vi "CSM Module.vi"(7 "Name (\"\" to Use UUID)":string="CSM Tiny") -> ()   [LabVIEW 2017]
uses:
  src/user.lib/_NEVSTOP/Communicable State Machine(CSM)/AdvanceAPI/CSM - Revert Arguments-Safe String.vi
  src/user.lib/_NEVSTOP/Communicable State Machine(CSM)/AdvanceAPI/CSM - Make String Arguments Safe.vi
  src/user.lib/_NEVSTOP/Communicable State Machine(CSM)/AdvanceAPI/CSM - Break Down Multiple States String.vi
  src/user.lib/_NEVSTOP/Communicable State Machine(CSM)/AdvanceAPI/CSM - Compact Multiple States.vi
  src/user.lib/_NEVSTOP/Communicable State Machine(CSM)/AdvanceAPI/CSM - Keywords.vi
  src/user.lib/_NEVSTOP/Communicable State Machine(CSM)/_Shared/Trim Single-line Text.vi
  src/user.lib/_NEVSTOP/Communicable State Machine(CSM)/Communicable State Machine.lvlib
panel:
  out "State History":string
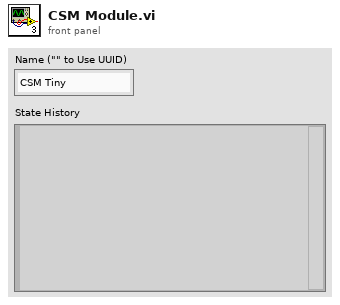
[diagram p1: front panel]
types:
  T1 = enum32{"Invalid", "Standard", "Closed", "Hidden", "Minimized", "Maximized"}
  T2 = enum32{"invalid app kind", "Development System", "Run Time System", "Student Edition", "Embedded LabVIEW", "Evaluation", "Custom"}
  T3 = typedef "Communicable State Machine.lvlib/_CSM_Response Source Message.ctl" = cluster{"‘State":string, "’Arguments":string, "’Error":errorcluster}
  T4 = cluster{"Current VI Reference":refnum<vi>, "Close Panel on Exit?":bool}
  T5 = cluster{"Core":cluster{"Current VI Reference":refnum<vi>, "Close Panel on Exit?":bool}, "Your Boolean data":bool, "Your string data":string}
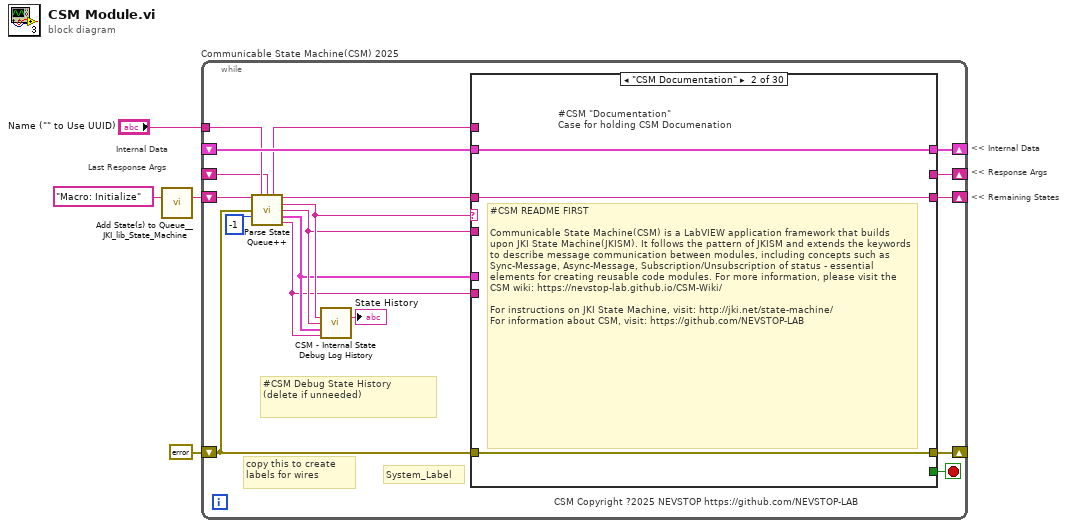
[diagram p0: block diagram]
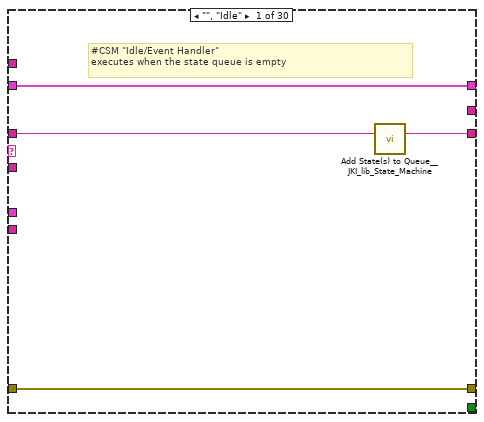
[diagram p2: hidden frame]
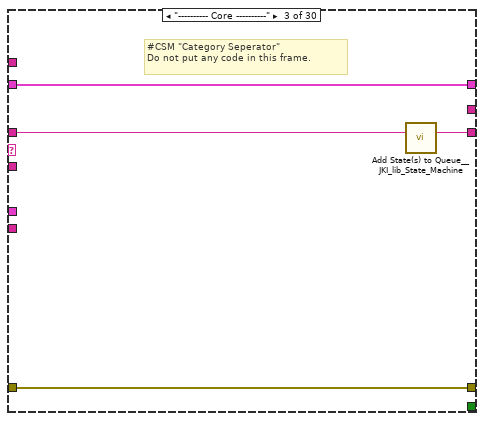
[diagram p3: hidden frame]
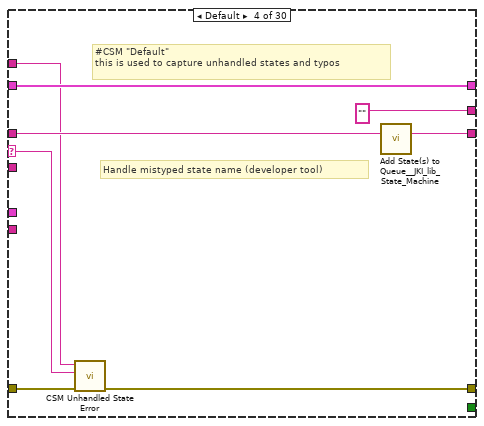
[diagram p4: hidden frame]
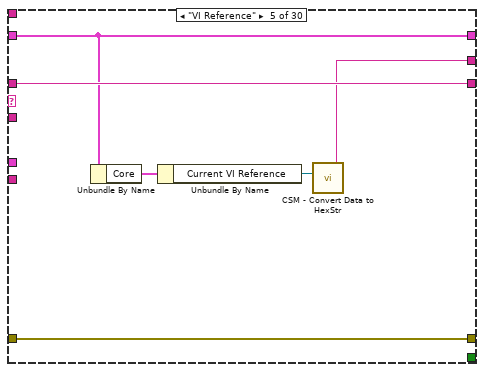
[diagram p5: hidden frame]
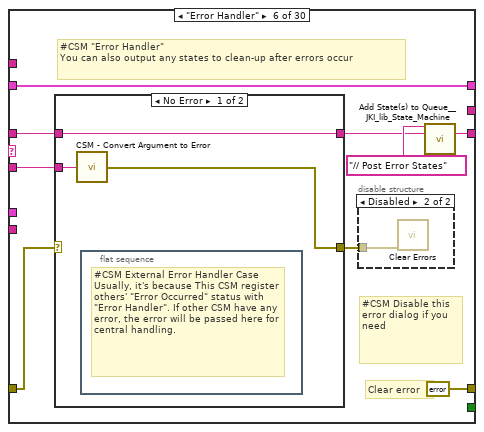
[diagram p6: hidden frame]
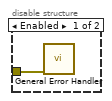
[diagram p7: hidden frame]
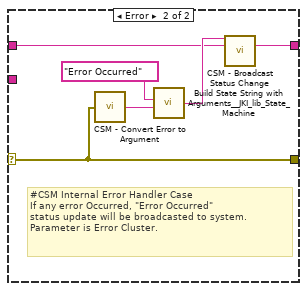
[diagram p8: hidden frame]
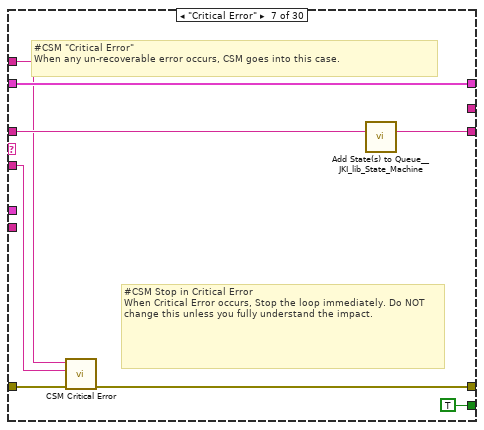
[diagram p9: hidden frame]
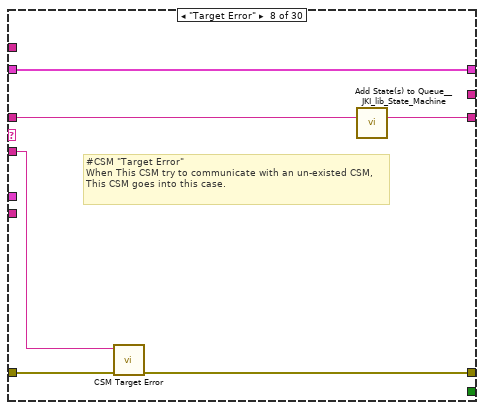
[diagram p10: hidden frame]
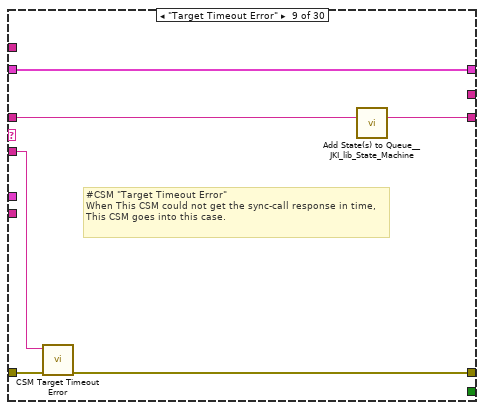
[diagram p11: hidden frame]
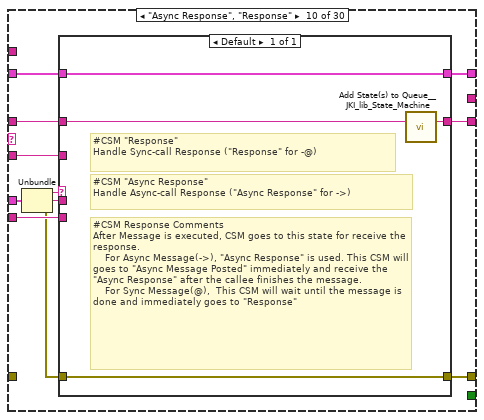
[diagram p12: hidden frame]
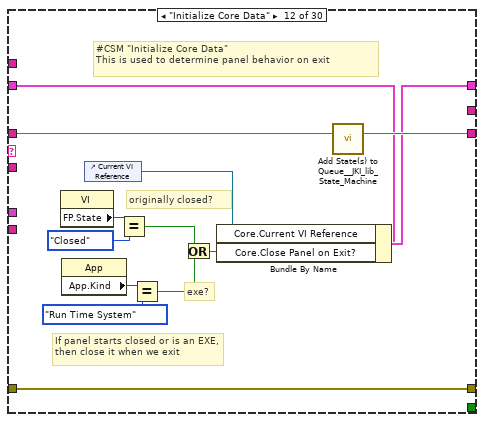
[diagram p14: hidden frame]
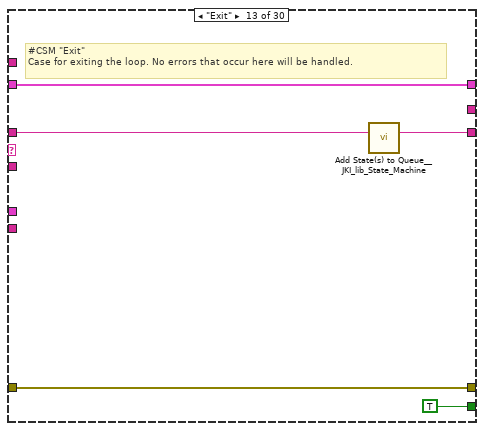
[diagram p15: hidden frame]
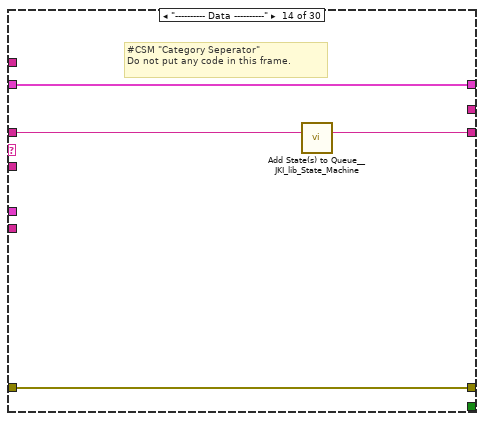
[diagram p16: hidden frame]
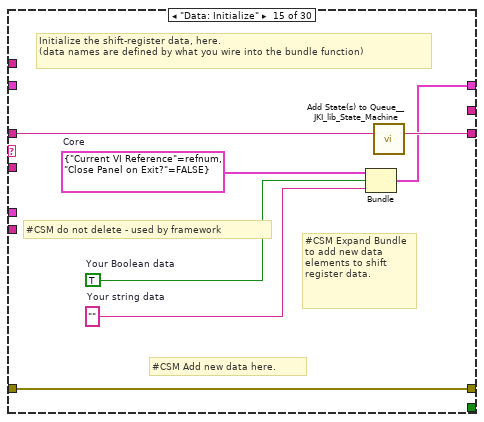
[diagram p17: hidden frame]
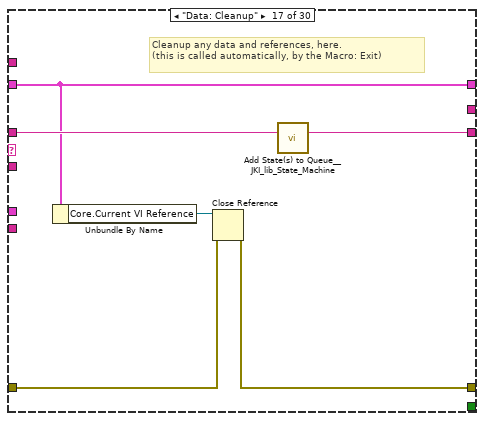
[diagram p19: hidden frame]
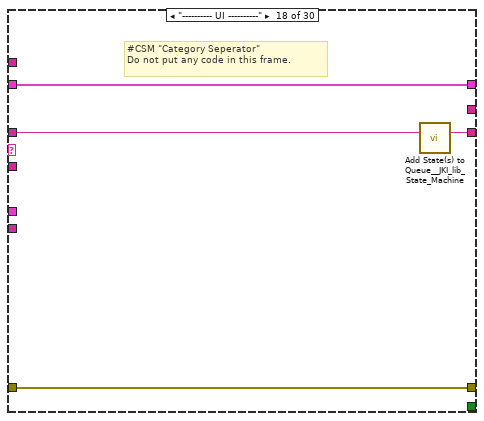
[diagram p20: hidden frame]
diagram:
  # "Last Response Args"
  # "Internal Data"
  # "<< Internal Data"
  # "<< Response Args"
  # "<< Remaining States"
  n1 = call <vilib>:"Add State(s) to Queue__JKI_lib_State_Machine.vi"("State(s) in (\"\")"="Macro: Initialize" ("Init State(\"Macro: Initialize\")")) -> ("States Out"=w4:string)  [unwired: 14 in]
  n2 = while "Communicable State Machine(CSM) 2025" {
    shift-right: [w17] -> _
    shift-left: _ -> [w16]
    shift-right: [w20] -> _
    shift-left: errorcluster {"status"=FALSE, "code"=0, "source"=""} ("error out") -> [w15]
    shift-right: [w19] -> _
    shift-left: w4 -> [w21]
    tunnel: "Name (\"\" to Use UUID)" -> [w13]
    shift-right: [w14] -> _
    shift-left: _ -> [w7]
    stop <- w18 stop-if-true
    # "#CSM Debug State History\n(delete if unneeded)"
    # "copy this to create labels for wires"
    # "System_Label"
    # "CSM Copyright ?2025 NEVSTOP https://github.com/NEVSTOP-LAB"
    n3 = call "Parse State Queue++.vi"("State Queue"=w21, "Name (\"\" to Use UUID)"=w13, "Response Arguments"=w7, "Previous Error"=w15, "Dequeue (1 ms)"=-1 ("Timeout")) -> ("Name Used"=w8:string, "Remaining States"=w22:string, "Current State"=w12:string, "Arguments"=w11:string, "Additional Information"=w10:T3, "Source CSM"=w9:string)  [unwired: 5 in]
    n4 = call "CSM - Internal State Debug Log History.vi"("State"=w12, "Arguments (\"\")"=w11, ">> Response Source Message >>"=w10, "Source (\"\")"=w9) -> ("Debug Log"=→"State History":string)  [unwired: 11 in]
    n5 = case shown="\"CSM Documentation\"" w12 {
      selector: w12 -> [_ _ _ w36 _ _ _ _ _ _ _ _ _ _ _ _ _ _ _ _ _ _ _ _ _ _ _ _ _ _]
      tunnel: w22 -> [w23 w28 w33 w40 w46 w52 w73 w79 w85 w93 w104 w118 w123 w127 w134 w136 w143 w147 w151 w157 w172 w241 w246 w253 w255 w259 w264 w271 w275 w279]
      tunnel: w11 -> [_ _ _ _ _ w51 w69 w78 w83 w92 _ _ _ _ _ _ _ _ _ w152 w166 _ _ _ _ _ w262 _ _ _]
      tunnel: w16 -> [w24 w27 w30 w38 w45 w55 w74 w80 w86 w95 w103 w111 w121 w124 _ w135 w138 w144 w149 w155 w168 w238 w243 w250 w254 w258 w263 w268 w272 w276]
      tunnel: [w25 w29 w31 w34 w47 errorcluster {"status"=FALSE, "code"=0, "source"=""} ("error out") w70 w76 w82 w98 w105 w115 w120 w125 w131 w137 w139 w145 w148 w153 w169 w239 w244 w251 w256 w260 w265 w269 w273 w277] -> w20
      tunnel: w15 -> [w25 w29 w31 w41 w47 w53 w75 w77 w84 _ w105 w115 w120 w125 w131 w137 w140 w145 w148 w154 w170 w239 w244 w251 w256 w260 w265 w269 w273 w277]
      tunnel: [w26 w28 w32 w39 w46 w48 w72 w81 w87 w94 w104 w117 w122 w126 w133 w136 w142 w146 w150 w156 w171 w240 w245 w252 w255 w259 w264 w270 w274 w278] -> w19
      tunnel: [_ _ _ _ _ _ TRUE _ _ _ _ _ TRUE _ _ _ _ _ _ _ _ _ _ _ _ _ _ _ _ _] -> w18
      tunnel: [w24 w27 w30 w38 w45 w55 w74 w80 w86 w96 w103 w116 w121 w124 w132 w135 w138 w144 w149 w155 w168 w238 w243 w250 w254 w258 w263 w268 w272 w276] -> w17
      tunnel: w9 -> [_ _ _ _ _ _ _ _ _ w90 _ _ _ _ _ _ _ _ _ _ _ _ _ _ _ _ _ _ _ _]
      tunnel: w10 -> [_ _ _ _ _ _ _ _ _ w97 _ _ _ _ _ _ _ _ _ _ _ _ _ _ _ _ _ _ _ _]
      tunnel: [_ _ _ "" w42 _ _ _ _ _ _ _ _ _ _ _ _ _ _ _ _ _ _ _ _ "API1 Response" w261 _ _ _] -> w14
      tunnel: w8 -> [_ _ _ w35 _ _ w68 _ _ _ _ _ _ _ _ _ _ _ _ _ _ _ _ _ _ _ _ _ _ _]
      frame "", "Idle" {
        # "#CSM \"Idle/Event Handler\"\nexecutes when the state queue is empty"
        n6 = call <vilib>:"Add State(s) to Queue__JKI_lib_State_Machine.vi"("State(s) in (\"\")"=w23) -> ("States Out"=w26:string)  [unwired: 14 in]
      }
      frame "CSM Documentation" {
        # "#CSM README FIRST\n\nCommunicable State Machine(CSM) is a LabVIEW application framework that builds upon JKI State Machine(JKISM). It follows the pattern of JKISM and extends the keywords to describe message communication between modules, including concepts such as Sync-Message, Async-Message, Subscription/Unsubscription of status - essential elements for creating reusable code modules. For more information, please visit the CSM wiki: https://nevstop-lab.github.io/CSM-Wiki/\n\nFor instructions on JKI State Machine, visit: http://jki.net/state-machine/\nFor information about CSM, visit: https://github.com/NEVSTOP-LAB"
        # "#CSM \"Documentation\"\nCase for holding CSM Documenation"
      }
      frame "---------- Core ----------" {
        # "#CSM \"Category Seperator\"\nDo not put any code in this frame."
        n7 = call <vilib>:"Add State(s) to Queue__JKI_lib_State_Machine.vi"("State(s) in (\"\")"=w33) -> ("States Out"=w32:string)  [unwired: 14 in]
      }
      frame Default {
        # "#CSM \"Default\"\nthis is used to capture unhandled states and typos"
        # "Handle mistyped state name (developer tool)"
        n8 = call "CSM Unhandled State Error.vi"("error in (no error)"=w41, "Undefined State"=w36, "CSM Name"=w35) -> ("error out"=w34:errorcluster)  [unwired: 8 in]
        n9 = call <vilib>:"Add State(s) to Queue__JKI_lib_State_Machine.vi"("State(s) in (\"\")"=w40) -> ("States Out"=w39:string)  [unwired: 14 in]
      }
      frame "VI Reference" {
        n10 = Unbundle By Name(w45) -> ("Core"=w44:T4)
        n11 = Unbundle By Name(w44) -> ("Current VI Reference"=w43:refnum<vi>)
        n12 = call "CSM - Convert Data to HexStr.vi"("Variant"=w43) -> ("HEX String (0-9,A-F)"=w42:string)  [unwired: 8 in]
      }
      frame "Error Handler" {
        # "#CSM Disable this error dialog if you need"
        # "#CSM \"Error Handler\"\nYou can also output any states to clean-up after errors occur"
        # "Clear error"
        n13 = case shown="No Error" w53 {
          selector: w53 -> [_ w62]
          tunnel: [w61 w64] -> w49
          tunnel: w52 -> [w61 w63]
          tunnel: w51 -> [w60 _]
          tunnel: [w59 w62] -> w54
          frame No Error {
            n14 = call "CSM - Convert Argument to Error.vi"("Argument"=w60) -> ("Error"=w59:errorcluster)  [unwired: 4 in]
            n15 = flat-sequence {
              frame #0 {
                # "#CSM External Error Handler Case\nUsually, it's because This CSM register others' \"Error Occurred\" status with \"Error Handler\". If other CSM have any error, the error will be passed here for central handling."
              }
            }
          }
          frame Error {
            # "#CSM Internal Error Handler Case \nIf any error Occurred, \"Error Occurred\" \nstatus update will be broadcasted to system.\nParameter is Error Cluster."
            n16 = call "CSM - Convert Error to Argument.vi"("Error"=w62) -> ("Argument"=w66:string)  [unwired: 4 in]
            n17 = call <vilib>:"Build State String with Arguments__JKI_lib_State_Machine.vi"("Arguments (\"\")"=w66, "State"="Error Occurred" ("Status with Arguments")) -> ("State with Arguments"=w65:string)  [unwired: 4 in]
            n18 = call "CSM - Broadcast Status Change.vi"("Status With Arguments"=w65, "State Queue"=w63) -> ("Remaining States"=w64:string)  [unwired: 13 in]
          }
        }
        n19 = disable-structure shown="Disabled" {
          disable-tunnel: w54 -> [w57 w58]
          frame Enabled {
            n20 = call <vilib>:"General Error Handler.vi"("error in (no error)"=w57) -> ()  [unwired: 10 in, 5 out]
          }
          frame Disabled {
            n21 = call <vilib>:"Clear Errors.vi"("error in (no error)"=w58) -> ()  [unwired: 5 in, 2 out]
          }
        }
        n22 = call <vilib>:"Add State(s) to Queue__JKI_lib_State_Machine.vi"("State(s) in Front (\"\")"="// Post Error States", "State(s) in (\"\")"=w49) -> ("States Out"=w48:string)  [unwired: 13 in]
      }
      frame "Critical Error" {
        # "#CSM Stop in Critical Error\nWhen Critical Error occurs, Stop the loop immediately. Do NOT change this unless you fully understand the impact."
        # "#CSM \"Critical Error\"\nWhen any un-recoverable error occurs, CSM goes into this case."
        n23 = call "CSM Critical Error.vi"("error in (no error)"=w75, "Arugments (As Reason)"=w69, "CSM Name"=w68) -> ("error out"=w70:errorcluster)  [unwired: 8 in]
        n24 = call <vilib>:"Add State(s) to Queue__JKI_lib_State_Machine.vi"("State(s) in (\"\")"=w73) -> ("States Out"=w72:string)  [unwired: 14 in]
      }
      frame "Target Error" {
        # "#CSM \"Target Error\"\nWhen This CSM try to communicate with an un-existed CSM, This CSM goes into this case."
        n25 = call "CSM Target Error.vi"("error in (no error)"=w77, "Arguments (As CSM Name)"=w78) -> ("error out"=w76:errorcluster)  [unwired: 9 in]
        n26 = call <vilib>:"Add State(s) to Queue__JKI_lib_State_Machine.vi"("State(s) in (\"\")"=w79) -> ("States Out"=w81:string)  [unwired: 14 in]
      }
      frame "Target Timeout Error" {
        # "#CSM \"Target Timeout Error\"\nWhen This CSM could not get the sync-call response in time, This CSM goes into this case."
        n27 = call "CSM Target Timeout Error.vi"("error in (no error)"=w84, "Arguments (As CSM Name)"=w83) -> ("error out"=w82:errorcluster)  [unwired: 9 in]
        n28 = call <vilib>:"Add State(s) to Queue__JKI_lib_State_Machine.vi"("State(s) in (\"\")"=w85) -> ("States Out"=w87:string)  [unwired: 14 in]
      }
      frame "Async Response", "Response" {
        n29 = Unbundle(w97) -> ("‘State"=w91:string, "’Arguments"=w89:string, "’Error"=w88:errorcluster)
        n30 = case shown="Default" w91 {
          tunnel: [w102] -> w98
          tunnel: w88 -> [w102]
          tunnel: [w101] -> w96
          tunnel: w95 -> [w101]
          tunnel: [w99] -> w94
          tunnel: w93 -> [w100]
          tunnel: w92 -> [_]
          tunnel: w90 -> [_]
          tunnel: w89 -> [_]
          frame Default {
            # "#CSM Response Comments\nAfter Message is executed, CSM goes to this state for receive the response.\n    For Async Message(->), \"Async Response\" is used. This CSM will goes to \"Async Message Posted\" immediately and receive the \"Async Response\" after the callee finishes the message.\n    For Sync Message(@),  This CSM will wait until the message is done and immediately goes to \"Response\""
            # "#CSM \"Async Response\"\nHandle Async-call Response (\"Async Response\" for ->)"
            # "#CSM \"Response\"\nHandle Sync-call Response (\"Response\" for -@)"
            n31 = call <vilib>:"Add State(s) to Queue__JKI_lib_State_Machine.vi"("State(s) in (\"\")"=w100) -> ("States Out"=w99:string)  [unwired: 14 in]
          }
        }
      }
      frame "Async Message Posted" {
        # "#CSM \"Async Message Posted\"\nAfter Async Message is posted (-> or ->| ), CSM goes to this state for post-action.\nYou can use Argument - State to tell which Async Message is called."
      }
      frame "Initialize Core Data" {
        # "#CSM \"Initialize Core Data\"\nThis is used to determine panel behavior on exit"
        # "originally closed?"
        # "exe?"
        # "If panel starts closed or is an EXE, then close it when we exit"
        n32 = property class="VI"() -> ("FP.State"=w108:T1)  [unwired: 2 in, 2 out]
        n33 = property class="App"() -> ("App.Kind"=w114:T2)  [unwired: 2 in, 2 out]
        n34 = control-ref of="Current VI Reference"() -> (w109:refnum<vi>)
        n35 = Equal?(x=w108, y=T1."Closed" ("Front Panel Window:State")) -> (x = y?=w106:bool)
        n36 = Equal?(x=w114, y=T2."Run Time System" ("Application:Kind")) -> (x = y?=w112:bool)
        n37 = Or(x=w106, y=w112) -> (x .or. y?=w110:bool)
        n38 = Bundle By Name(cluster=w111, "Core.Current VI Reference"=w109, "Core.Close Panel on Exit?"=w110) -> (w116:T5)
        n39 = call <vilib>:"Add State(s) to Queue__JKI_lib_State_Machine.vi"("State(s) in (\"\")"=w118) -> ("States Out"=w117:string)  [unwired: 14 in]
      }
      frame "Exit" {
        # "#CSM \"Exit\"\nCase for exiting the loop. No errors that occur here will be handled."
        n40 = call <vilib>:"Add State(s) to Queue__JKI_lib_State_Machine.vi"("State(s) in (\"\")"=w123) -> ("States Out"=w122:string)  [unwired: 14 in]
      }
      frame "---------- Data ----------" {
        # "#CSM \"Category Seperator\"\nDo not put any code in this frame."
        n41 = call <vilib>:"Add State(s) to Queue__JKI_lib_State_Machine.vi"("State(s) in (\"\")"=w127) -> ("States Out"=w126:string)  [unwired: 14 in]
      }
      frame "Data: Initialize" {
        w128 = T4 {"Current VI Reference"=refnum, "Close Panel on Exit?"=FALSE}  # Core
        w130 = TRUE  # Your Boolean data
        w129 = ""  # Your string data
        # "#CSM do not delete - used by framework"
        # "#CSM Expand Bundle to add new data elements to shift register data."
        # "#CSM Add new data here."
        # "Initialize the shift-register data, here.\n(data names are defined by what you wire into the bundle function)"
        n42 = Bundle("Core"=w128, "Your Boolean data"=w130, "Your string data"=w129) -> (w132:T5)  [unwired: 1 in]
        n43 = call <vilib>:"Add State(s) to Queue__JKI_lib_State_Machine.vi"("State(s) in (\"\")"=w134) -> ("States Out"=w133:string)  [unwired: 14 in]
      }
      frame "Data: Update Indicators" {
      }
      frame "Data: Cleanup" {
        # "Cleanup any data and references, here.\n(this is called automatically, by the Macro: Exit)"
        n44 = Unbundle By Name(w138) -> ("Core.Current VI Reference"=w141:refnum<vi>)
        n45 = Close Reference(reference=w141, error in (no error)=w140) -> (error out=w139:errorcluster)
        n46 = call <vilib>:"Add State(s) to Queue__JKI_lib_State_Machine.vi"("State(s) in (\"\")"=w143) -> ("States Out"=w142:string)  [unwired: 14 in]
      }
      frame "---------- UI ----------" {
        # "#CSM \"Category Seperator\"\nDo not put any code in this frame."
        n47 = call <vilib>:"Add State(s) to Queue__JKI_lib_State_Machine.vi"("State(s) in (\"\")"=w147) -> ("States Out"=w146:string)  [unwired: 14 in]
      }
      frame "UI: Initialize" {
        # "#CSM \"UI: Initialize\"\nInitialize the User Interface, here.\n(this is called automatically, by the Macro: Init)"
        n48 = call <vilib>:"Add State(s) to Queue__JKI_lib_State_Machine.vi"("State(s) in (\"\")"=w151) -> ("States Out"=w150:string)  [unwired: 14 in]
      }
      frame "UI: Cursor Set" {
        # "#CSM \"UI: Cursor Set\"\nSet and Unset Cursor Busy.\n(Usage: \"UI: Cursor Set >> Busy|Idle\")"
        # "Argument"
        n49 = disable-structure shown="TARGET_TYPE!=Windows" {
          disable-tunnel: w154 -> [w160 w165]
          disable-tunnel: [w159 w165] -> w153
          disable-tunnel: w152 -> [w158 _]
          frame condition #0 (active) {
            n50 = case shown="\"Idle\", Default" w158 {
              tunnel: w160 -> [w162 w164]
              tunnel: [w161 w163] -> w159
              frame "Idle", Default {
                n51 = call <vilib>:"Unset Busy.vi"("error in (no error)"=w162) -> ("error out"=w161:errorcluster)  [unwired: 10 in]
              }
              frame "Busy" {
                n52 = call <vilib>:"Set Busy.vi"("error in (no error)"=w164) -> ("error out"=w163:errorcluster)  [unwired: 9 in, 1 out]
              }
            }
          }
          frame condition #1 {
          }
        }
        n53 = call <vilib>:"Add State(s) to Queue__JKI_lib_State_Machine.vi"("State(s) in (\"\")"=w157) -> ("States Out"=w156:string)  [unwired: 14 in]
      }
      frame "UI: Front Panel State" {
        # "#CSM \"UI: Front Panel State\"\nSet Front Panel Open or Closed\n(Usage: \"UI: Front Panel State >> Open|Close\")"
        # "Argument"
        n54 = Unbundle By Name(w168) -> ("Core.Current VI Reference"=w167:refnum<vi>)
        n55 = call <vilib>:"Add State(s) to Queue__JKI_lib_State_Machine.vi"("State(s) in (\"\")"=w172) -> ("States Out"=w171:string)  [unwired: 14 in]
        n56 = case shown="\"Close\", \"Closed\"" w166 {
          tunnel: w170 -> [w178 w193 w204 w217 w230]
          tunnel: [w180 w194 w206 w219 w232] -> w169
          tunnel: w167 -> [w179 w191 w205 w218 w231]
          frame "Open", "Standard", Default {
            w173 = T1."Standard" ("State")
            n57 = property class="VI"(reference=w179, error in=w178) -> (reference out=w176:refnum<vi>, error out=w177:errorcluster, "FP.State"=w175:T1)
            n58 = Not Equal?(x=w175, y=w173) -> (x != y?=w174:bool)
            n59 = case shown="True" w174 {
              tunnel: [w184 w186] -> w180
              tunnel: w177 -> [w183 w186]
              tunnel: w176 -> [w182 _]
              tunnel: w173 -> [w181 _]
              frame True {
                n60 = invoke class="VI" method="FP.Open"(reference=w182, error in=w183, "Activate"=TRUE, "State"=w181) -> (error out=w184:errorcluster)  [unwired: 1 in, 4 out]
              }
              frame False {
              }
            }
          }
          frame "Close", "Closed" {
            n61 = property class="VI"(reference=w191, error in=w193) -> (reference out=w190:refnum<vi>, error out=w192:errorcluster, "FP.State"=w188:T1)
            n62 = Not Equal?(x=w188, y=T1."Closed" ("Front Panel Window:State")) -> (x != y?=w187:bool)
            n63 = case shown="False" w187 {
              tunnel: [w195 w198] -> w194
              tunnel: w192 -> [w195 w197]
              tunnel: w190 -> [_ w196]
              frame False {
              }
              frame True {
                n64 = invoke class="VI" method="FP.Close"(reference=w196, error in=w197) -> (error out=w198:errorcluster)  [unwired: 1 in, 2 out]
              }
            }
          }
          frame "Hidden", "Hide" {
            w199 = T1."Hidden" ("State")
            n65 = property class="VI"(reference=w205, error in=w204) -> (reference out=w202:refnum<vi>, error out=w203:errorcluster, "FP.State"=w201:T1)
            n66 = Not Equal?(x=w201, y=w199) -> (x != y?=w200:bool)
            n67 = case shown="True" w200 {
              tunnel: [w210 w211] -> w206
              tunnel: w203 -> [w209 w211]
              tunnel: w202 -> [w208 _]
              tunnel: w199 -> [w207 _]
              frame True {
                n68 = invoke class="VI" method="FP.Open"(reference=w208, error in=w209, "State"=w207) -> (error out=w210:errorcluster)  [unwired: 2 in, 4 out]
              }
              frame False {
              }
            }
          }
          frame "Minimize", "Minimized" {
            w212 = T1."Minimized" ("State")
            n69 = property class="VI"(reference=w218, error in=w217) -> (reference out=w215:refnum<vi>, error out=w216:errorcluster, "FP.State"=w214:T1)
            n70 = Not Equal?(x=w214, y=w212) -> (x != y?=w213:bool)
            n71 = case shown="True" w213 {
              tunnel: [w223 w224] -> w219
              tunnel: w216 -> [w222 w224]
              tunnel: w215 -> [w221 _]
              tunnel: w212 -> [w220 _]
              frame True {
                n72 = invoke class="VI" method="FP.Open"(reference=w221, error in=w222, "State"=w220) -> (error out=w223:errorcluster)  [unwired: 2 in, 4 out]
              }
              frame False {
              }
            }
          }
          frame "Maximize", "Maximized" {
            w225 = T1."Maximized" ("State")
            n73 = property class="VI"(reference=w231, error in=w230) -> (reference out=w228:refnum<vi>, error out=w229:errorcluster, "FP.State"=w227:T1)
            n74 = Not Equal?(x=w227, y=w225) -> (x != y?=w226:bool)
            n75 = case shown="True" w226 {
              tunnel: [w236 w237] -> w232
              tunnel: w229 -> [w235 w237]
              tunnel: w228 -> [w234 _]
              tunnel: w225 -> [w233 _]
              frame True {
                n76 = invoke class="VI" method="FP.Open"(reference=w234, error in=w235, "State"=w233) -> (error out=w236:errorcluster)  [unwired: 2 in, 4 out]
              }
              frame False {
              }
            }
          }
        }
      }
      frame "---------- Macro ----------" {
        # "#CSM \"Category Seperator\"\nDo not put any code in this frame."
        n77 = call <vilib>:"Add State(s) to Queue__JKI_lib_State_Machine.vi"("State(s) in (\"\")"=w241) -> ("States Out"=w240:string)  [unwired: 14 in]
      }
      frame "Macro: Initialize" {
        # "#CSM \"Macro: Initialize\"\nInitialization Macro (This is called once, when the VI starts)"
        n78 = call <vilib>:"Add State(s) to Queue__JKI_lib_State_Machine.vi"("State(s) in Front (\"\")"="Data: Initialize\nInitialize Core Data\nData: Update Indicators", "State(s) in (\"\")"=w246) -> ("States Out"=w245:string)  [unwired: 13 in]
      }
      frame "Macro: Exit" {
        # "#CSM \"Macro: Exit\"\nExit Macro (This is called once, when the VI exits)"
        n79 = call <vilib>:"Add State(s) to Queue__JKI_lib_State_Machine.vi"("State(s) in Front (\"\")"="//Exit Sub-Modules ", "State(s) at Back (\"\")"="Data: Cleanup\nExit") -> ("States Out"=w248:string)  [unwired: 13 in]
        n80 = call <vilib>:"Add State(s) to Queue__JKI_lib_State_Machine.vi"("State(s) in Front (\"\")"=w248, "State(s) in (\"\")"=w253) -> ("States Out"=w252:string)  [unwired: 13 in]
      }
      frame "---------- API ----------" {
        # "#CSM \"Category Seperator\"\nDo not put any code in this frame."
      }
      frame "API: API1" {
        # "#CSM API Example\nCopy/Rename this case for your own API"
        # "#CSM Response\nConnect this to return the response of your API"
        # "#CSM >> Msg/Rep's CSM >>\nIf you need to tell who triggered this state , use this string. If it's this case itself, this string is \"\"."
        # "#CSM >> Arguments >>\nDeal with the parameter if any"
      }
      frame "API: API2" {
        # "#CSM API Example\nCopy/Rename this case for your own API"
        # "unpack Hex String  to Variant\nif complex parameter is needed."
        n81 = call "CSM - Convert HexStr to Data.vi"("HEX String"=w262) -> ()  [unwired: 7 in, 2 out]
        n82 = disable-structure shown="Disabled" {
          disable-tunnel: [w266 "API2 Response"] -> w261
          frame Disabled {
            # "pack variant to hexstr \nif complex response is needed."
            # "complex Response"
            n83 = call "CSM - Convert Data to HexStr.vi"() -> ("HEX String (0-9,A-F)"=w266:string)  [unwired: 9 in]
          }
          frame Enabled {
          }
        }
      }
      frame "---------- Action ----------" {
        # "#CSM \"Category Seperator\"\nDo not put any code in this frame."
        n84 = call <vilib>:"Add State(s) to Queue__JKI_lib_State_Machine.vi"("State(s) in (\"\")"=w271) -> ("States Out"=w270:string)  [unwired: 14 in]
      }
      frame "Action: action1" {
        # "#CSM \"Internal State\"\nThis category is used for holding internal states"
        n85 = call <vilib>:"Add State(s) to Queue__JKI_lib_State_Machine.vi"("State(s) in (\"\")"=w275) -> ("States Out"=w274:string)  [unwired: 14 in]
      }
      frame "Action: action2" {
        # "#CSM \"Internal State\"\nThis category is used for holding internal states"
        n86 = call <vilib>:"Add State(s) to Queue__JKI_lib_State_Machine.vi"("State(s) in (\"\")"=w279) -> ("States Out"=w278:string)  [unwired: 14 in]
      }
    }
  }
